vi "Call.vi"(6 "Error":errorcluster, 10 "Msg":T1 {"Metadata"."AbsoluteTime" format="%<%x %.3X>T"}, 11 "Actor":refnum<class "Actor.lvclass">) -> (2 "Msg":T1 {"Metadata"."AbsoluteTime" format="%<%x %.3X>T"}, 3 "Actor":refnum<class "Actor.lvclass">, 4 "Error":errorcluster)   [LabVIEW 2020, in "_Template.lvlib" / "{{Msg}}.lvlib"]
uses:
  {{Msg}}.lvlib
  Msg/Msg.lvclass
  jettl/jettl/jettl.lvlib
  jettl/jettl/Actor/Actor.lvclass
  jettl/jettl/Lifecycle.ctl
  jettl/jettl/Metadata.ctl
  Msg.ctl
  jettl/jettl/Metadata/Metadata.lvclass
  jettl/jettl/Origin.ctl
panel:
  # "This front panel should not be manipulated."
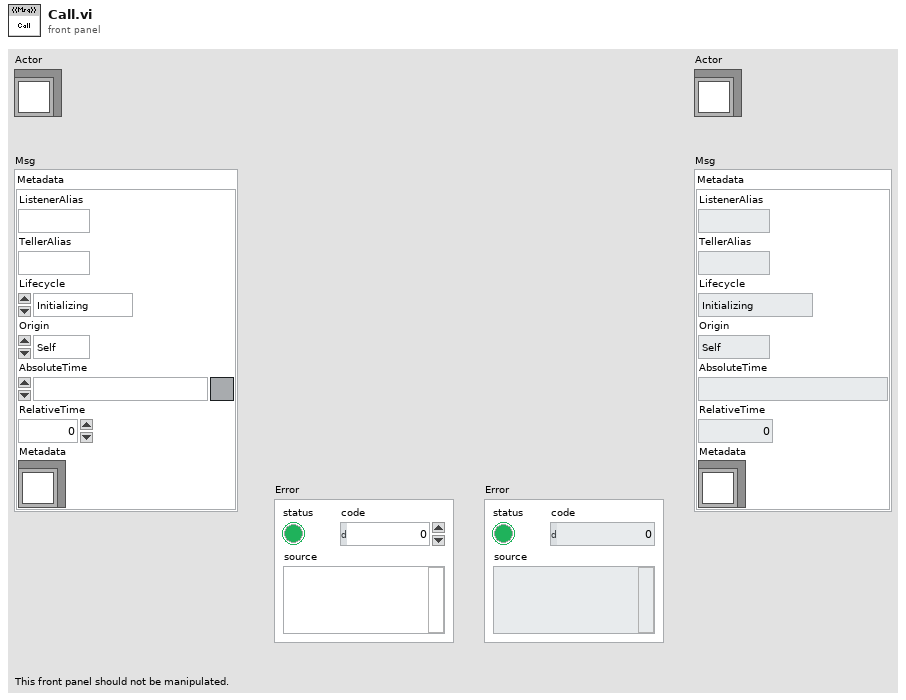
[diagram p1: front panel]
types:
  T1 = typedef "_Template.lvlib/{{Msg}}.lvlib/Msg.ctl" = cluster{"Metadata":T2}
  T2 = typedef "jettl.lvlib/Metadata.ctl" = cluster{"ListenerAlias":string, "TellerAlias":string, "Lifecycle":T3, "Origin":T4, "AbsoluteTime":timestamp, "RelativeTime":dbl, "Metadata":refnum<class "Metadata.lvclass">}
  T3 = typedef "jettl.lvlib/Lifecycle.ctl" = enum16{"Initializing", "SettingUp", "Starting", "Running", "Stopping", "TearingDown", "Terminated"}
  T4 = typedef "jettl.lvlib/Origin.ctl" = enum16{"Self", "Parent", "Child"}
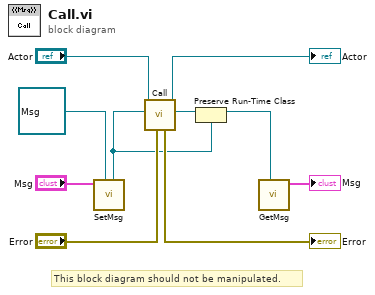
[diagram p0: block diagram]
diagram:
  # "This block diagram should not be manipulated."
  n1 = call "SetMsg.vi"(7:"Msg"=refnum<class "Msg.lvclass"> refnum ("_Template.lvlib:MessageTemplate.lvlib:{{Name}}.lvlib:ConcreteMessage.lvclass"), 11:"Msg"="Msg") -> ("Msg"=w1:refnum<class "Msg.lvclass">)  [unwired: 9 in]
  n2 = call "Call.vi"("Error"="Error", "Message"=w1, "Actor"="Actor") -> ("Message"=w5:refnum<class "Message.lvclass">, "Actor"=→"Actor":refnum<class "Actor.lvclass">, "Error"=→"Error":errorcluster)  [unwired: 6 in]
  n3 = Preserve Run-Time Class(object in=w5, 2:w1) -> (object out=w4:refnum<class "Msg.lvclass">)  [unwired: 1 in, 1 out]
  n4 = call "GetMsg.vi"("Message"=w4) -> ("PayloadCluster"=→"Msg":T1)  [unwired: 10 in]
